vi "WriteResetPositionToZero.vi"(8 "error in":errorcluster, 11 "VISA resource name":refnum<visa-resource-name>) -> (0 "error out":errorcluster, 3 "VISA resource name out":refnum<visa-resource-name>)   [LabVIEW 2019, in "Mark 10 TSTM-DC.lvlib"]
uses:
  Mark 10 TSTM-DC.lvlib
  Mark 10 Event Monitor/Mark 10 Event Monitor.lvlib
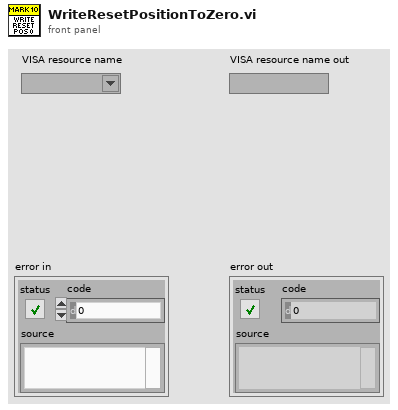
[diagram p1: front panel]
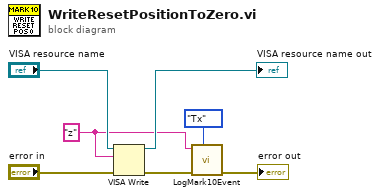
[diagram p0: block diagram]
diagram:
  w2 = "z" ("write buffer")
  n1 = VISA Write(VISA resource name="VISA resource name", write buffer=w2, error in (no error)="error in") -> (VISA resource name out=→"VISA resource name out":refnum<visa-resource-name>, error out=w5:errorcluster)  [unwired: 1 out]
  n2 = call "LogMark10Event.vi"("Type"=enum16{"Tx", "Rx"}."Tx", "Error In"=w5, "Event"=w2) -> ("Error Out"=→"error out":errorcluster)  [unwired: 8 in]
